vi "Get Null Parameters.vi"(8 "error in (no error)":errorcluster, 11 "Null Adapter in":refnum<class "Null Adapter.lvclass">) -> (0 "error out":errorcluster, 3 "Null Adapter out":refnum<class "Null Adapter.lvclass">)   [LabVIEW 2018, in "Null Adapter.lvlib" / "Null Adapter.lvclass"]
uses:
  Null Adapter.lvclass
  c:/Sequence Automation/Plugins/Measurement Interface.lvlibp/Measurement Interface.lvclass
  Plugins/Measurement Interface.lvlibp/Private Methods/Measurement Parameters/Read Measurement Parameters.vi
  Plugins/String Database.lvlibp/String Database.lvclass
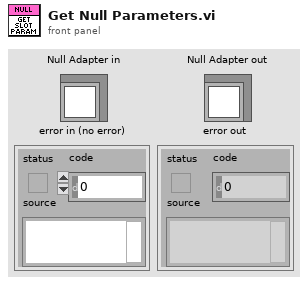
[diagram p1: front panel]
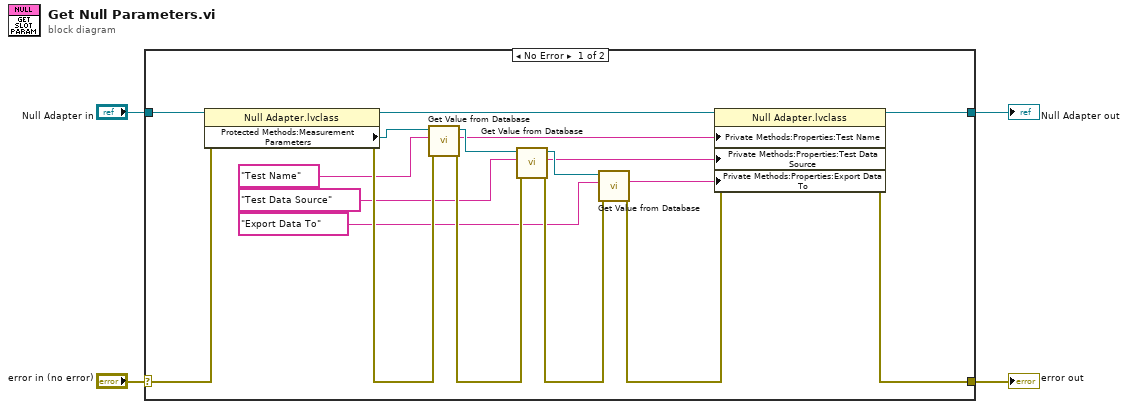
[diagram p0: block diagram]
diagram:
  n1 = case shown="No Error" "error in (no error)" {
    selector: "error in (no error)" -> [w22 w24]
    tunnel: [w18 w24] -> w3
    tunnel: [w17 w23] -> w1
    tunnel: "Null Adapter in" -> [w21 w23]
    frame No Error {
      n2 = property class="Null Adapter.lvclass"(reference=w21, error in=w22) -> (reference out=w5:refnum<class "Null Adapter.lvclass">, error out=w19:errorcluster, "Protected Methods:Measurement Parameters"=w20:refnum<class "String Database.lvclass">)
      n3 = call "Get Value from Database.vi"("error in (no error)"=w19, "Entry Name"="Test Name", "Message in"=w20) -> ("error out"=w15:errorcluster, "Entry Value"=w8:string, "Message out"=w16:refnum<class "String Database.lvclass">)  [unwired: 5 in, 1 out]
      n4 = call "Get Value from Database.vi"("error in (no error)"=w15, "Entry Name"="Test Data Source", "Message in"=w16) -> ("error out"=w13:errorcluster, "Entry Value"=w7:string, "Message out"=w11:refnum<class "String Database.lvclass">)  [unwired: 5 in, 1 out]
      n5 = call "Get Value from Database.vi"("error in (no error)"=w13, "Entry Name"="Export Data To", "Message in"=w11) -> ("error out"=w12:errorcluster, "Entry Value"=w6:string)  [unwired: 5 in, 2 out]
      n6 = property class="Null Adapter.lvclass"(reference=w5, error in=w12, "Private Methods:Properties:Test Name"=w8, "Private Methods:Properties:Test Data Source"=w7, "Private Methods:Properties:Export Data To"=w6) -> (reference out=w17:refnum<class "Null Adapter.lvclass">, error out=w18:errorcluster)
    }
    frame Error {
    }
  }
  "error out" <- w3
  "Null Adapter out" <- w1
